vi "Handle Command.vi"(8 "error in":errorcluster, 10 "Load New Speaker Chirp in":refnum<class "Load New Speaker Chirp.lvclass">, 11 "Object In":refnum<class>) -> (0 "error out":errorcluster, 1 "Command Successful?":bool, 2 "Load New Speaker Chirp Out":refnum<class "Load New Speaker Chirp.lvclass">, 3 "Object Out":refnum<class>)   [LabVIEW 2014, in "ePAS Library.lvlib" / "Load New Speaker Chirp.lvclass"]
doc: "Load a new speaker tophat. The tophat is a broadband \"chirp\" that allows the caller to characterize te acoustic properties of the cavity (retrieve Q and f0)."
uses:
  Load New Speaker Chirp.lvclass
  Instrument/ePAS.lvclass
  FPGA/Session/Exscalabar FPGA.lvclass
  Instrument/ePAS.lvclass/ePAS.ctl
  Load New Speaker Chirp.lvclass/Load New Speaker Chirp.ctl
  reusable/PAS/Main/PAS.lvclass/PAS.ctl
  FPGA/Session/Exscalabar FPGA.lvclass/Exscalabar FPGA.ctl
  FPGA/Session/Read Ex FPGA Ref.vi
  <vilib>/Utility/error.llb/Error Cluster From Error Code.vi
  <vilib>/rvi/errors/niLvFpgaAdjustHostInterfaceError.vi
  FPGA/R FPGA Ref.ctl
  <vilib>/rvi/interface/nirviMethod/nirviMethod.xnode
  FPGA Bitfiles/FPGA Server.lvbitx
  reusable/PAS/Main/PAS.lvclass
  ePAS Library.lvlib
  <vilib>/FPGAPlugInAG/PXI-7842R/niLvFpga_WriteFifo_PXI-7842R.vi
  <vilib>/rvi/errors/niLvFpgaMergeErrorWithErrorCode.vi
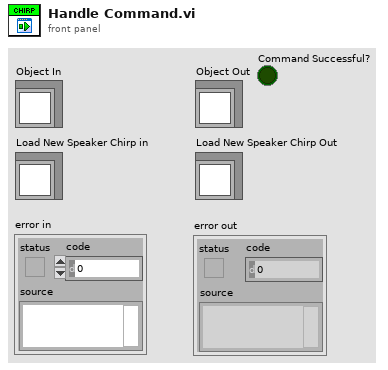
[diagram p1: front panel]
types:
  T1 = typedef "Session - Root.lvclass/Session Handle.ctl" = refnum<data-value>
  T2 = typedef "ePAS Library.lvlib/R FPGA Ref.ctl" = refnum<k20>
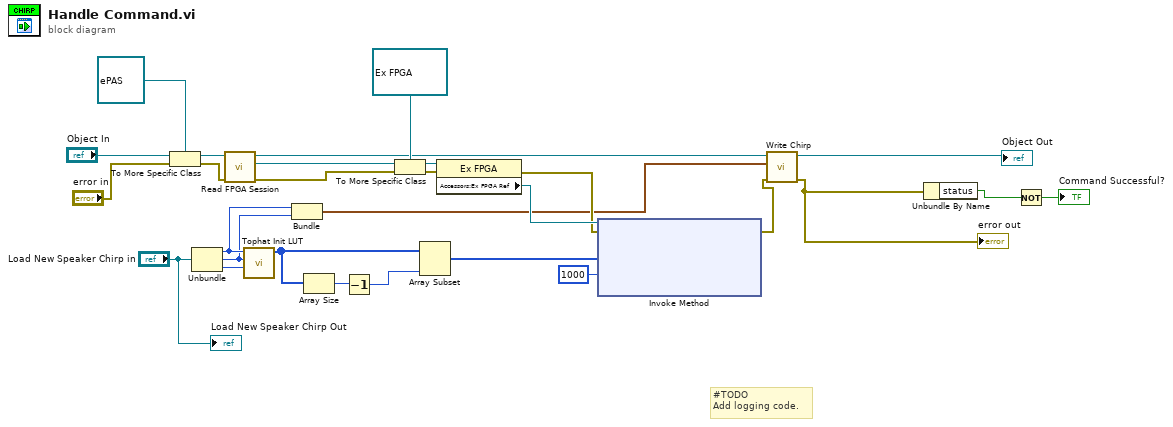
[diagram p0: block diagram]
diagram:
  # "#TODO\nAdd logging code."
  n1 = To More Specific Class(target class=refnum<class "ePAS.lvclass"> refnum ("ePAS.lvclass"), reference="Object In", error in="error in") -> (specific class reference=w25:refnum<class "ePAS.lvclass">, error out=w11:errorcluster)
  n2 = Unbundle("Load New Speaker Chirp in") -> (w6:i16, w5:i16, w28:i32)
  n3 = call "Read FPGA Session.vi"("error in (no error)"=w11, "ePAS in"=w25) -> ("error out"=w13:errorcluster, "Session Handle"=w23:T1, "ePAS out"=w10:refnum<class "ePAS.lvclass">)  [unwired: 7 in]
  n4 = call "Tophat Init LUT.vi"("Number of  Elements"=w28, "Df"=w5, "f0"=w6) -> ("Init Data Out"=w18:i16[])  [unwired: 6 in]
  n5 = Bundle("fcenter"=w6, "bandwidth"=w5) -> (w7:cluster{"fcenter":i16, "bandwidth":i16})  [unwired: 1 in]
  n6 = Array Size(array=w18) -> (size(s)=w17:i32)
  n7 = Decrement(x=w17) -> (x-1=w16:i32)
  n8 = To More Specific Class(target class=refnum<data-value> refnum ("Session Handle"), reference=w23, error in=w13) -> (specific class reference=w21:refnum<data-value>, error out=w20:errorcluster)
  n9 = Array Subset(array=w18, length=w16) -> (w14:i16[])  [unwired: 1 in]
  n10 = property class="Ex FPGA"(reference=w21, error in=w20) -> (error out=w12:errorcluster, "Accessors:Ex FPGA Ref"=w19:T2)  [unwired: 1 out]
  n11 = xnode "Invoke Method"("FPGA VI Reference In"=w19, "error in"=w12, "Data"=w14, "Timeout (ms)"=1000) -> ("error out"=w9:errorcluster)  [unwired: 2 out]
  n12 = call "Write Chirp.vi"("error in (no error)"=w9, "Chirp"=w7, "PAS in"=w10) -> ("error out"=w3:errorcluster, "PAS out"=→"Object Out":refnum<class "ePAS.lvclass">)  [unwired: 7 in]
  "error out" <- w3
  n13 = Unbundle By Name(w3) -> ("status"=w2:bool)
  n14 = Not(x=w2) -> (.not. x?=→"Command Successful?":bool)
  "Load New Speaker Chirp Out" <- "Load New Speaker Chirp in"
